vi "FGV_Indicator.vi"(7 "Action":T3, 11 "Indicator Data In":T1={"相機、光源"={"相機選擇"=0, "光源選擇"=0, "光源亮度"=0}, "Session Out"="cam1", "Cam#Light#Strength"=""} {"相機、光源"."光源亮度" step=1 scale=0.0..255.0; "相機、光源"."相機選擇" items=["相機 1", "相機 2", "相機 3", "相機 4", "相機 5", "相機 6", "相機 7", "相機 8"]; "相機、光源"."光源選擇" items=["光源 1", "光源 2", "光源 3", "光源 4", "光源 5", "光源 6", "光源 7", "光源 8"]}) -> (3 "Indicator Data Out":T1={"相機、光源"={"相機選擇"=0, "光源選擇"=0, "光源亮度"=0}, "Session Out"="cam0", "Cam#Light#Strength"=""} {"相機、光源"."光源亮度" step=1 scale=0.0..255.0; "相機、光源"."相機選擇" items=["相機 1", "相機 2", "相機 3", "相機 4", "相機 5", "相機 6", "相機 7", "相機 8"]; "相機、光源"."光源選擇" items=["光源 1", "光源 2", "光源 3", "光源 4", "光源 5", "光源 6", "光源 7", "光源 8"]})   [LabVIEW 2015]
uses:
  control/Control_Indicator Action(FGV).ctl
  control/Control_Indicator(FGV) #.ctl
  <vilib>/userdefined/High Color/IMAQdx.ctl
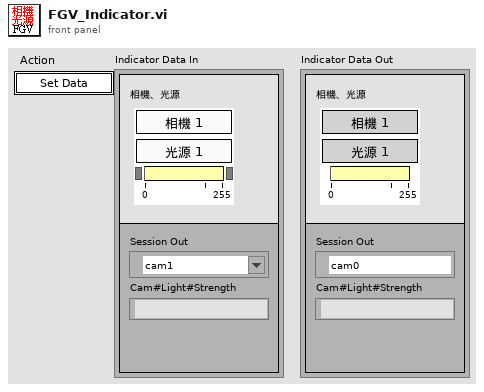
[diagram p1: front panel]
types:
  T1 = typedef "Control_Indicator(FGV) #.ctl" = cluster{"相機、光源":cluster{"相機選擇":u8, "光源選擇":u16, "光源亮度":u8}, "Session Out":T2, "Cam#Light#Strength":string}
  T2 = typedef "IMAQdx.ctl" = refnum<k21>
  T3 = typedef "Control_Indicator Action(FGV).ctl" = enum16{"Set Data", "Get Data", "Idle"}
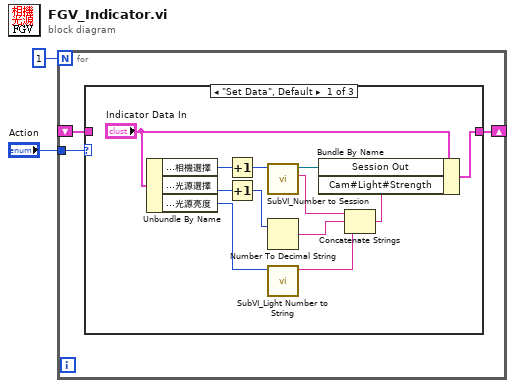
[diagram p0: block diagram]
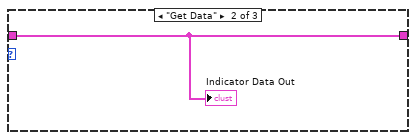
[diagram p2: hidden frame]
diagram:
  n1 = for {
    N: 1 -> [_]
    tunnel: "Action" -> [w5]
    shift-right: [w4] -> _
    shift-left: _ -> [w3]
    n2 = case shown="\"Set Data\", Default" w5 {
      tunnel: [w17 w18 w19] -> w4
      tunnel: w3 -> [_ w18 w19]
      frame "Set Data", Default {
        n3 = Unbundle By Name("Indicator Data In") -> ("相機、光源.相機選擇"=w8:u8, "相機、光源.光源選擇"=w10:u16, "相機、光源.光源亮度"=w15:u8)
        n4 = Increment(x=w8) -> (x+1=w7:u8)
        n5 = Increment(x=w10) -> (x+1=w9:u16)
        n6 = call "SubVI_Number to Session.vi"("Number"=w7) -> ("CCD#"=w11:string, "Session Out"=w16:T2)  [unwired: 9 in]
        n7 = Number To Decimal String(number=w9) -> (decimal integer string=w14:string)  [unwired: 1 in]
        n8 = call "SubVI_Light Number to String.vi"("Number"=w15) -> ("String"=w13:string)  [unwired: 10 in]
        n9 = Concatenate Strings(w11, w14, w13) -> (w12:string)
        n10 = Bundle By Name(cluster="Indicator Data In", "Session Out"=w16, "Cam#Light#Strength"=w12) -> (w17:T1)
      }
      frame "Get Data" {
        "Indicator Data Out" <- w18
      }
      frame "Idle" {
      }
    }
  }
